vi "Receiver_Example - 2 Channel - Experiment_12.vi"() -> ()   [LabVIEW 2022 SP3]
uses:
  <vilib>/httpClient/LabVIEWHTTPClient.lvlib
panel:
  out "BER LP3":dbl
  out "BER HP3":dbl
  out "Inst. BER LP - CH1":dbl format="%#_4g"
  out "OutputHPCH0":i8[](array[numeric])
  out "BER 16QAM":dbl
  out "LP - CH0":dbl format="%#_4g"
  in  "url 2":string="http://Cobot280-02.local:5000"
  out "Numeric":i32
  out "HP - CH0":dbl format="%#_4g"
  in  "url":string="http://Cobot280-01.local:5000"
  out "x = 0?":bool
  out "iterationsIM":dbl
  in  "State":i32
  in  "Counter":dbl
  in  "Tab Control 3":enum32{"OFDM - 4QAM", "16QAM"}(tab)
  in  "Switch mode":bool
  in  "Tab Control":T1(tab)
  in  "USRP ControledParameters":T2={"Active Antenna"="RX2", "Gain (dB)"=10.0, "Carrier Frequency"=2400000000.0, "IQ Rate"=2000000.0, "Active channels"="0,1"} {"IQ Rate" format="%#_6p"; "Carrier Frequency" format="%#_6p"; "Gain (dB)" format="%#_6f"}
  in  "Device selection":refnum<k15>="RIO0"
  in  "Trigger level":dbl=0.005 format="%f"
  out "CH0":T3
  out "CH1":T3
  out "SIG valid? - CH1":bool
  out "SIG valid? - CH0":bool
  out "Frequency offset - CH1":dbl
  out "Frequency offset - CH0":dbl
  out "Coerced Parameters":T4={"IQ Rate"=100000.0, "Carrier  Freq."=100000.0, "Gain"=0.0} {"Gain" format="%#_6f"; "Carrier  Freq." format="%#_6p"; "IQ Rate" format="%#_6p"}
  out "Error out":errorcluster
  out "Inst. BER HP - CH0":dbl format="%#_4g"
  out "Acc. BER HP - CH0":dbl format="%#_4g"
  out "Acum. Err HP - CH0":dbl
  out "No. Bits HP - CH0":dbl
  out "Acc. BER LP - CH0":dbl format="%#_4g"
  out "Inst. BER - CH1":dbl format="%#_4g"
  out "Inst. BER LP - CH0":dbl format="%#_4g"
  out "No. Bits - CH1":dbl
  out "No. Bits LP - CH0":dbl
  out "Acum. Err - CH1":dbl
  out "Acum. Err LP - CH0":dbl
  in  "Record BER":bool
  in  "Refresh Button":bool
  out "Acc. BER - CH1":dbl format="%#_4g"
  in  "Boolean 2":bool
  in  "Expected message HP - CH0":string="Critical Dataaaaa\nCritical Dataaaaa\nCritical Dataaaaa\nCritical Dataaaaa\nCritical Dataaaaa"
  out "Expected message HP Detected CH0":string="Non Critical Data\nNon Critical Data\nNon Critical Data\nNon Critical Data\nNon Critical Data"
  in  "Boolean 3":bool
  in  "Boolean":bool
  out "Expected message HP Detected CH1":string="Non Critical Data\nNon Critical Data\nNon Critical Data\nNon Critical Data\nNon Critical Data"
  out "Expected message LP Detected CH0":string="Non Critical Data\nNon Critical Data\nNon Critical Data\nNon Critical Data\nNon Critical Data"
  in  "Expected message - CH1":string="Critical Dataaaaa\nCritical Dataaaaa\nCritical Dataaaaa\nCritical Dataaaaa\nCritical Dataaaaa"
  in  "Expected message LP - CH0":string="Non Critical Data\nNon Critical Data\nNon Critical Data\nNon Critical Data\nNon Critical Data"
  in  "Boolean 5":bool
  in  "Expected message LP - CH1":string="Non Critical Data\nNon Critical Data\nNon Critical Data\nNon Critical Data\nNon Critical Data"
  out "Expected message LP Detected CH1":string="Non Critical Data\nNon Critical Data\nNon Critical Data\nNon Critical Data\nNon Critical Data"
  in  "High-Power Window Size":dbl=15.0 format="%#_6p"
  in  "Low-Power Window Size - CH0":dbl=15.0 format="%#_6p"
  in  "Threshold":dbl=10.0
  in  "Channel":bool
  in  "Expected message HP - CH0 2":string="Critical Dataaaaa\nCritical Dataaaaa\nCritical Dataaaaa\nCritical Dataaaaa\nCritical Dataaaaa\nNon Critical Data\nNon Critical Data\nNon Critical Data\nNon Critical Data\nNon Critical Data"
  in  "Tab Control 2":enum32{"1 Channel", "2 Channel"}(tab)
  in  "Save data 1 channel":bool
  out "Constellation Map 1 Channel":cdb[](graph)
  out "Low-Power BER - 1 Channel":dbl(graph)
  out "High-Power BER - 1 Channel":dbl(graph)
  out "High-Power Decoded message - 1 Channel":string
  out "Low-Power Decoded message - 1 Channel":string
  in  "Color Box":u32(colorbox)=11025761
  in  "Color Box 2":u32(colorbox)=7377308
  out "Low-Power Decoded message - CH0":string
  out "Decoded message - CH1":string
  out "Constellation Map 2 Channel":cluster{"Constellation":cdb[]}[](graph)
  out "Low-Power BER - 2 Channels":T5(graph)
  out "High-Power BER":T6(graph)
  out "High-Power Decoded message - CH0":string
  out "Low-Power Decoded message - CH1":string
  out "CH1 2":bool
  out "CH0 2":bool
  in  "Save data 2 channels":bool
  in  "Color Box 3":u32(colorbox)=11025761
  in  "Color Box 4":u32(colorbox)=7377308
  in  "Save data":bool
  out "Expected message  HP  Detected 2":string="Critical Dataaaaa\nCritical Dataaaaa\nCritical Dataaaaa\nCritical Dataaaaa\nCritical Dataaaaa"
  in  "Boolean 4":bool
  in  "High-Power Window Size 2":dbl=15.0 format="%#_6p"
  out "High-Power Instantaneous BER Graph 2":u8(slide) scale=0.0..100.0
  out "High-Power BER Graph 2":dbl(graph)
  out "No. Bits HP 2":dbl
  out "Acc. BER  HP 2":dbl format="%#_4g"
  out "Acum. Err HP 2":dbl
  out "Inst. BER HP 2":dbl format="%#_4g"
  in  "Expected message 2 HP 2":string="Critical Dataaaaa\nCritical Dataaaaa\nCritical Dataaaaa\nCritical Dataaaaa\nCritical Dataaaaa"
  out "High-Power Decoded Message 2":string
  in  "Record BER 2":bool
  out "Constellation Map 2":cdb[](graph)
  out "Frequency offset 2":dbl
  out "SIG valid? 2":bool
  in  "Refresh Button 2":bool
  out "Error out 2":errorcluster
  in  "error in (no error)":errorcluster
  # "OFDM Superposition Coded Receiver"
  # "Superposition coded\n(criticality-aware)"
  # "Single stream\n(criticality-agnostic)"
  # "1 Channel"
  # "2 Channel"
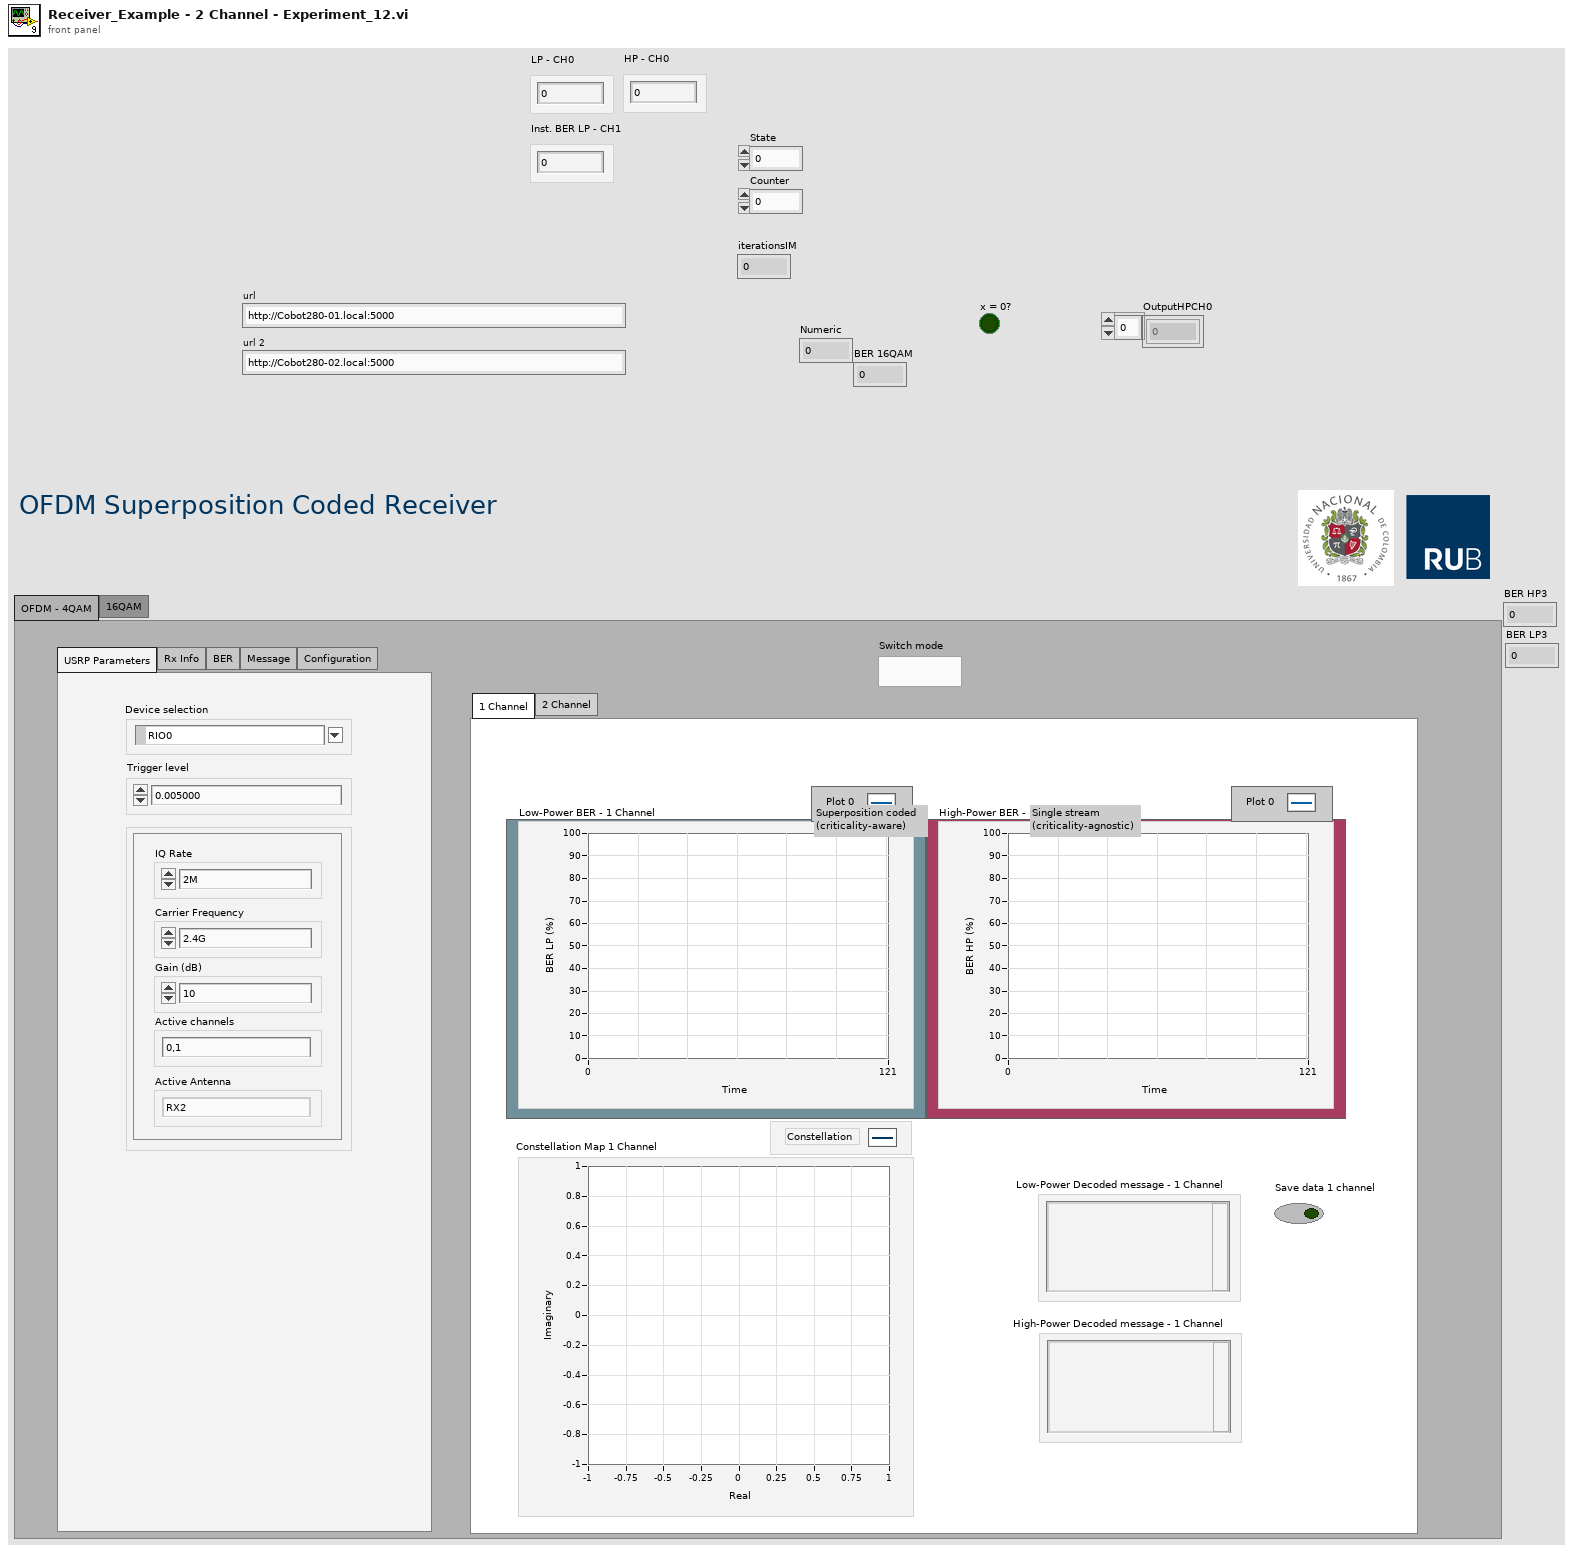
[diagram p1: front panel]
types:
  T1 = enum32{"USRP Parameters", "Rx Info", "BER", "Message", "Configuration"}
  T2 = cluster{"Active Antenna":string, "Gain (dB)":dbl, "Carrier Frequency":dbl, "IQ Rate":dbl, "Active channels":string}
  T3 = cluster{"Modulation type":enum16{"QPSK(4QAM)", "64QAM", "16QAM", "BPSK"}, "BCC rate (k/n)":enum16{"1/2", "2/3", "3/4"}}
  T4 = cluster{"IQ Rate":dbl, "Carrier  Freq.":dbl, "Gain":dbl}
  T5 = cluster{"Graph Instantaneous BER":dbl, "Graph Instantaneous BER":dbl, "Graph Instantaneous BER":dbl}
  T6 = cluster{"Graph Instantaneous BER":dbl, "Graph Instantaneous BER":dbl, "Inst. BER - CH1":dbl}
  T7 = enum16{"open", "replace", "create", "open or create", "replace or create", "replace or create with confirmation"}
  T8 = cluster{"coerced IQ rate":dbl, "coerced carrier frequency":dbl, "coerced gain":dbl}
  T9 = typedef "LabVIEWHTTPClient.lvlib/ClientHandle.ctl" = refnum<k1>
  T10 = typedef "angle_speed_def.ctl" = cluster{"degrees":dbl[], "speed":i32}
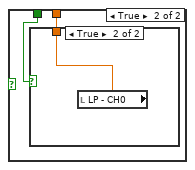
[diagram p2: hidden frame]
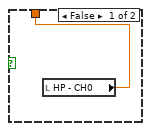
[diagram p3: hidden frame]
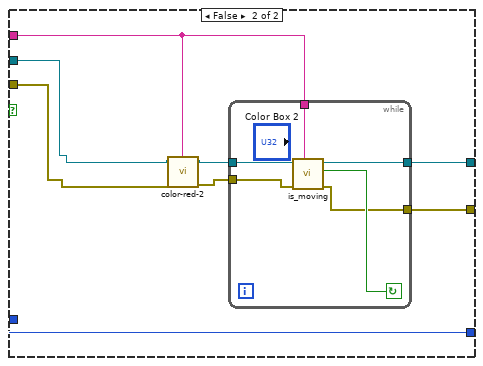
[diagram p4: hidden frame]
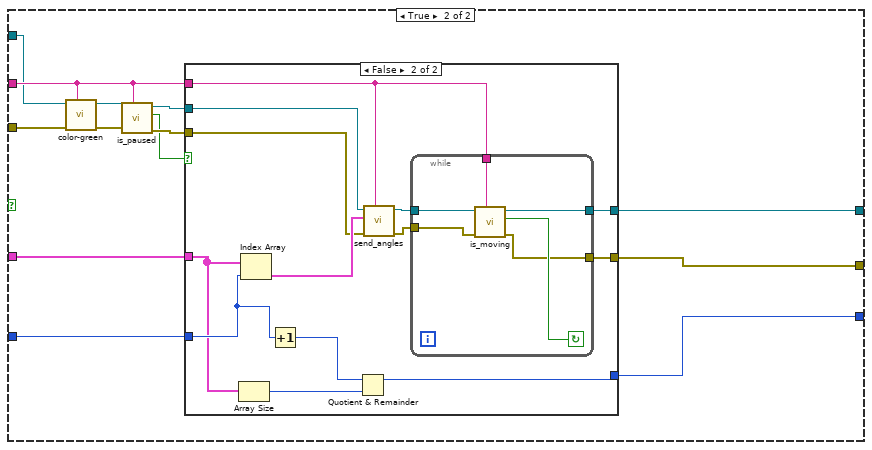
[diagram p5: hidden frame]
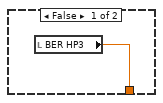
[diagram p7: hidden frame]
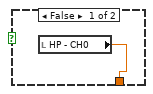
[diagram p8: hidden frame]
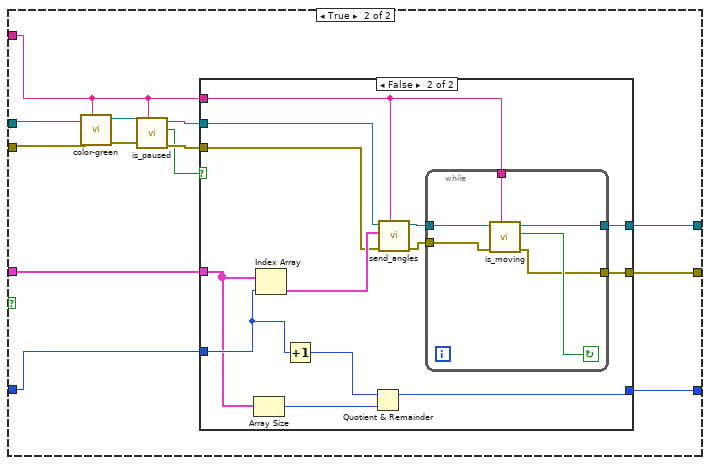
[diagram p10: hidden frame]
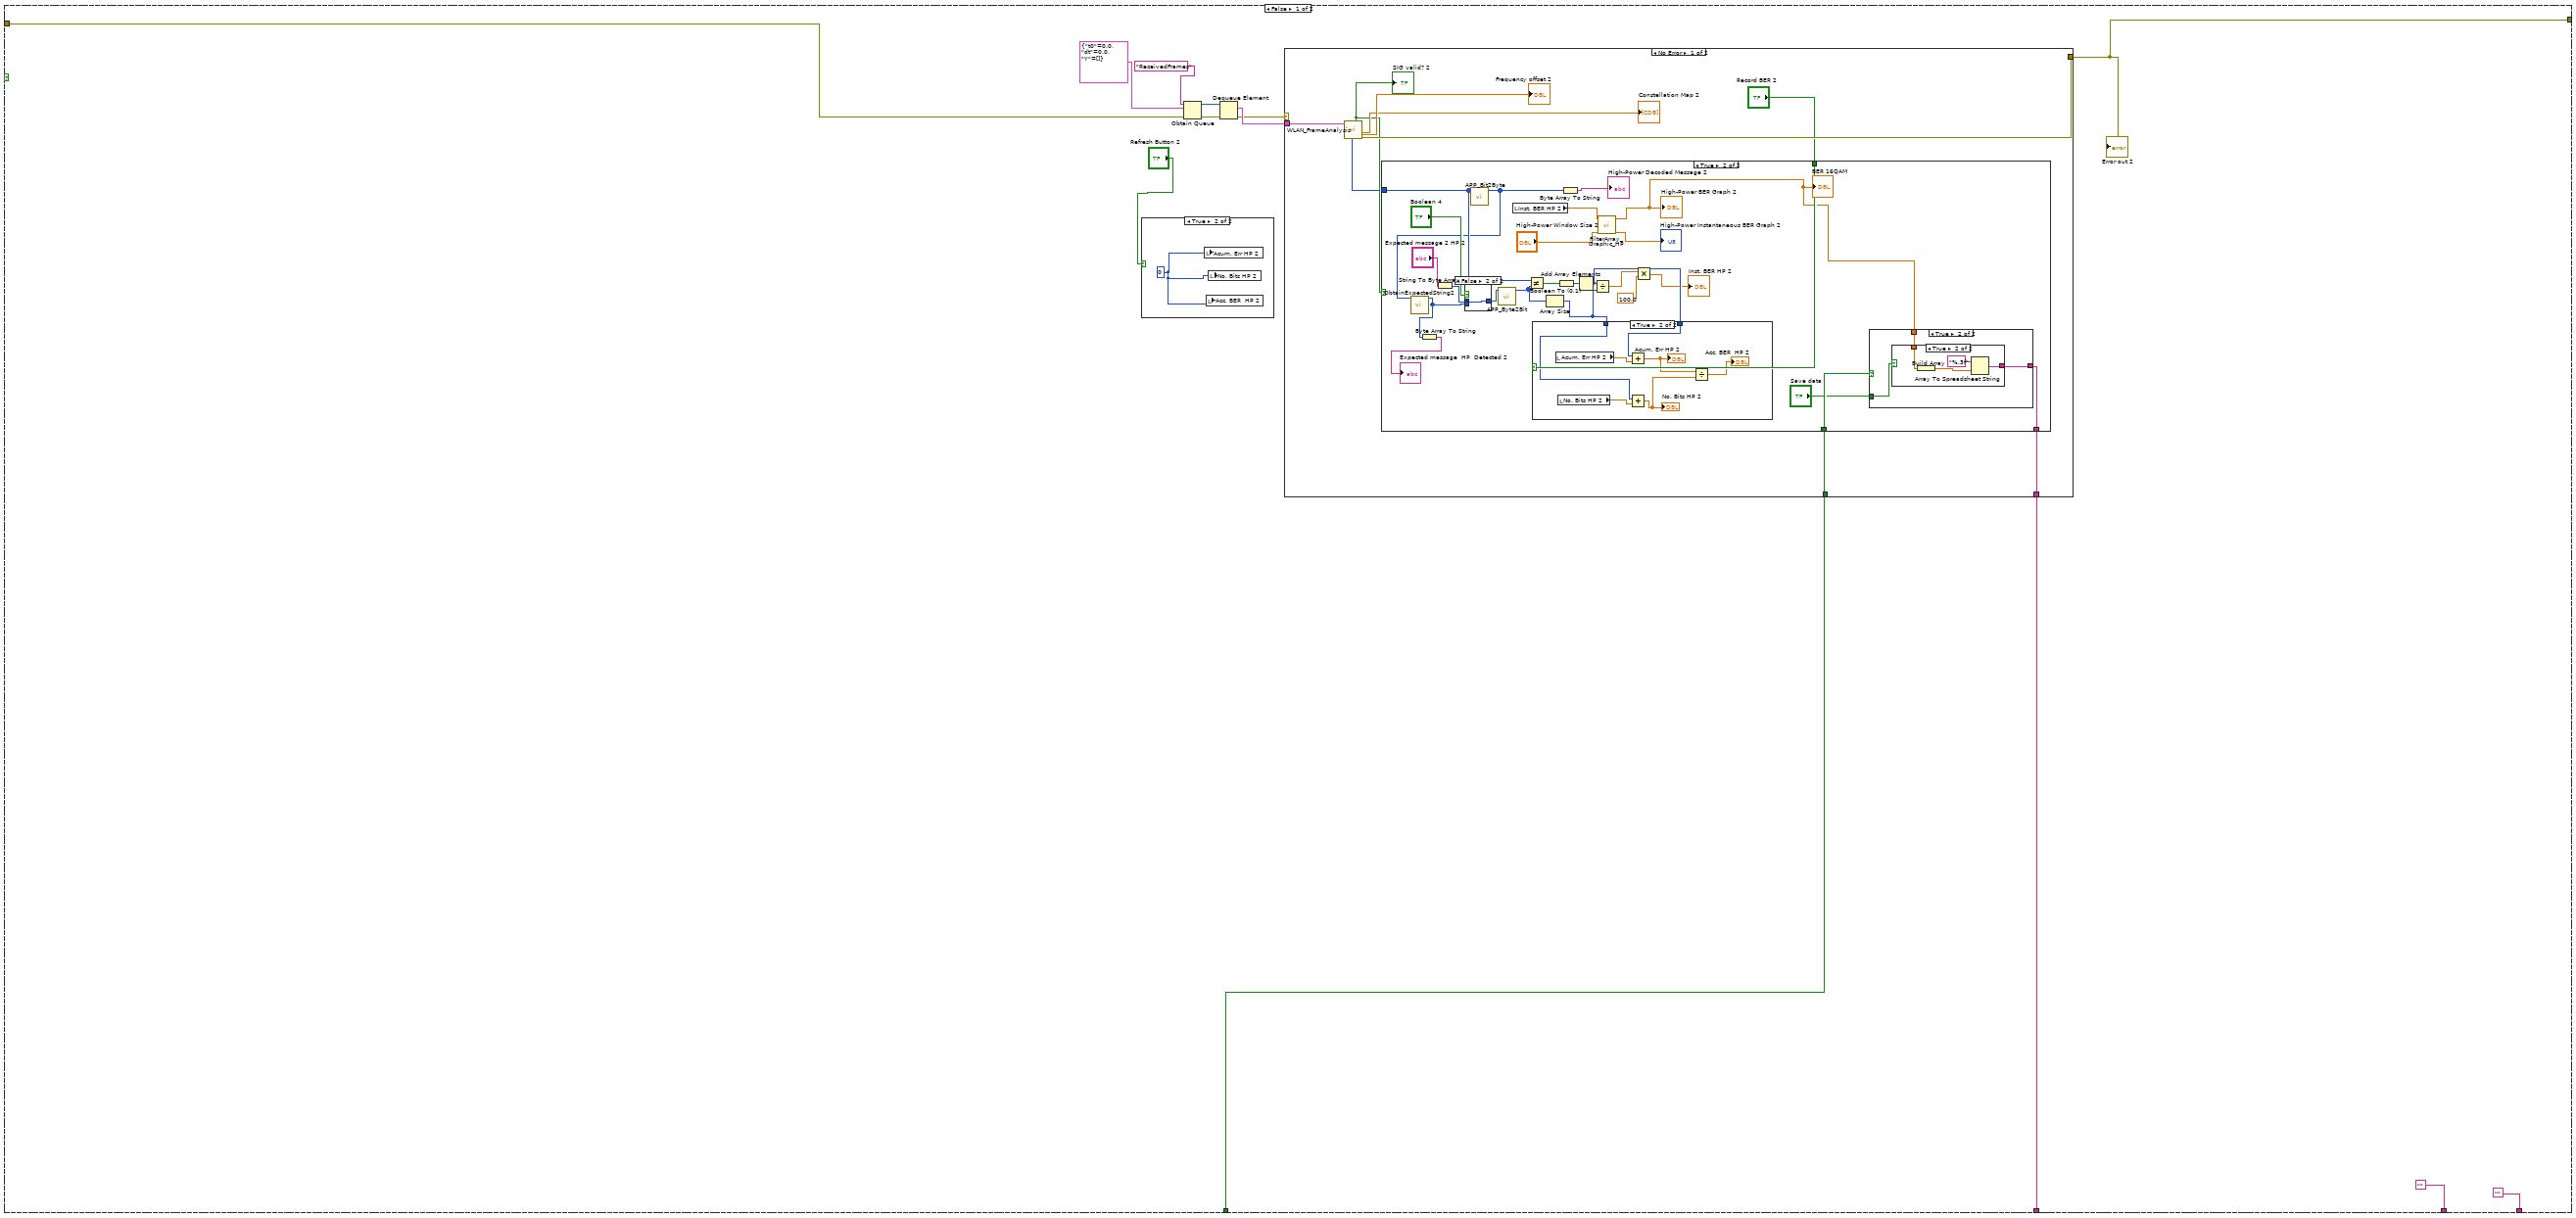
[diagram p12: hidden frame]
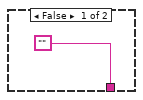
[diagram p14: hidden frame]
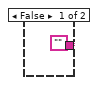
[diagram p15: hidden frame]
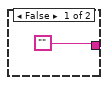
[diagram p16: hidden frame]
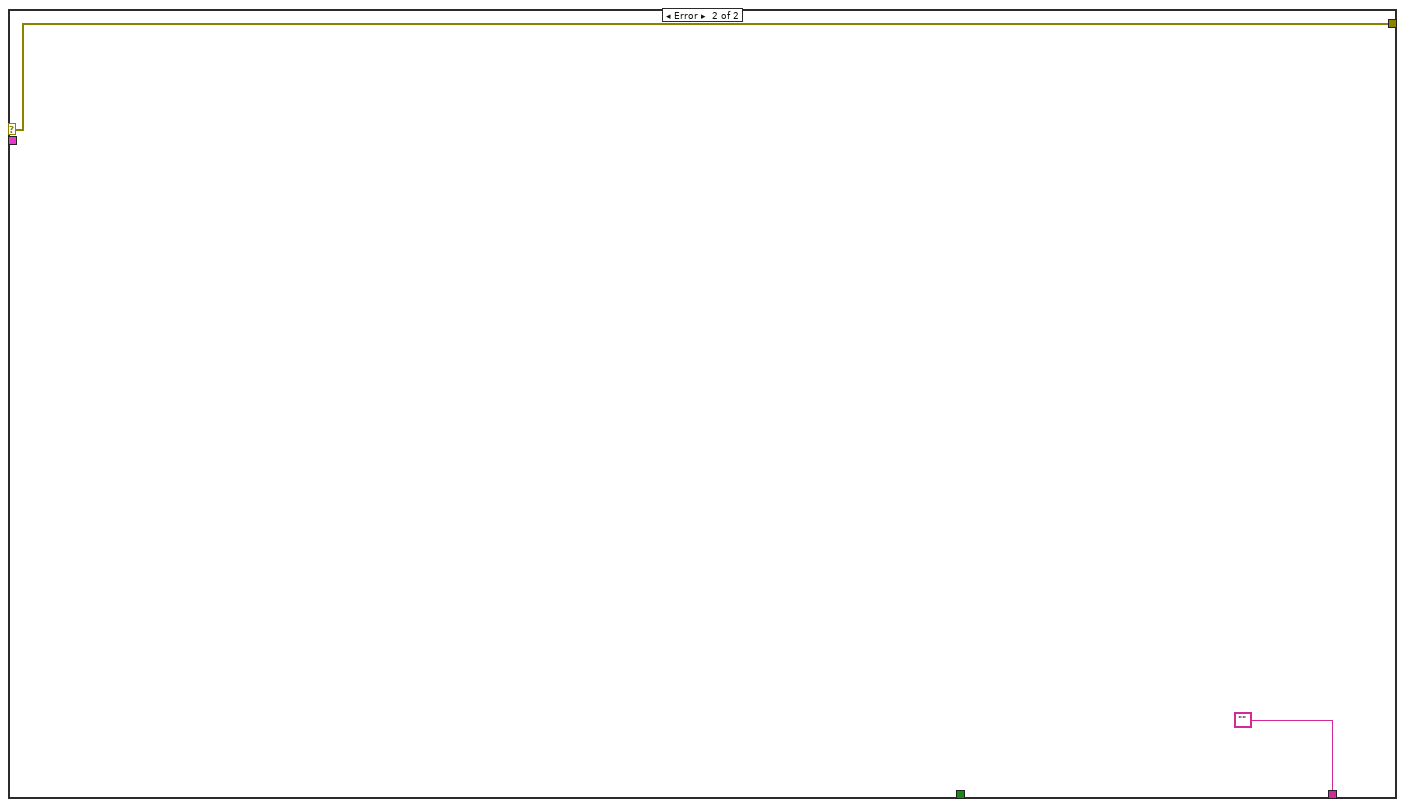
[diagram p19: hidden frame]
diagram:
  w23 = path "C:/Users/DKS/Desktop/Experiment/23_11_2023_with_graphs/12.10.2023/Supercoded Receiver with BER 12.10.2023/OFDM-Framework-LabVIEW-master/data"
  w45 = 0
  n1 = Build Path(base path=w23, name or relative path=path "data_OneChannel.txt" ("default name")) -> (appended path=w33:path)
  n2 = Build Path(base path=w23, name or relative path=path "data_16QAM.txt" ("default name")) -> (appended path=w43:path)
  n3 = Build Path(base path=w23, name or relative path=path "data_TwoChannels.txt" ("default name")) -> (appended path=w28:path)
  n4 = Delete(path (use dialog)=w33) -> (deleted path=w32:path)  [unwired: 4 in, 2 out]
  n5 = Delete(path (use dialog)=w43) -> (deleted path=w42:path)  [unwired: 4 in, 2 out]
  n6 = call "USRP_RXInit.vi"("device names"="Device selection", "USRP ControledParameters"="USRP ControledParameters", "error in (no error)"="error in (no error)") -> ("session handle out"=w48:refnum<k15>, "USRP CoercedParamters"=→"Coerced Parameters":T8, "error out"=w51:errorcluster)  [unwired: 5 in]
  n7 = Delete(path (use dialog)=w28) -> (deleted path=w27:path)  [unwired: 4 in, 2 out]
  n8 = Open/Create/Replace File(file path (use dialog)=w32, operation (0:open)=T7."create", access (0:read/write)=enum16{"read/write", "read-only", "write-only"}."write-only") -> (refnum out=w20:refnum<file>, error out=w19:errorcluster)  [unwired: 1 in, 3 out]
  n9 = Open/Create/Replace File(file path (use dialog)=w42, operation (0:open)=T7."create", access (0:read/write)=enum16{"read/write", "read-only", "write-only"}."write-only") -> (refnum out=w36:refnum<file>, error out=w37:errorcluster)  [unwired: 1 in, 3 out]
  n10 = Open/Create/Replace File(file path (use dialog)=w27, operation (0:open)=T7."create", access (0:read/write)=enum16{"read/write", "read-only", "write-only"}."write-only") -> (refnum out=w18:refnum<file>, error out=w17:errorcluster)  [unwired: 1 in, 3 out]
  n11 = call "WLAN_FrameCapture - 2 Channels.vi"("error in (no error)"=w51, "Trigger level"="Trigger level", "session handle"=w48) -> ()  [unwired: 8 in]
  n12 = while {
    tunnel: w51 -> [w77]
    tunnel: [w76] -> w49
    shift-right: [w71] -> w35
    shift-left: w37 -> [w69]
    shift-right: [w70] -> w34
    shift-left: w36 -> [w68]
    shift-right: [w65] -> w16
    shift-left: w20 -> [w66]
    shift-right: [w63] -> w15
    shift-left: w19 -> [w64]
    shift-right: [w59] -> w14
    shift-left: w18 -> [w62]
    shift-right: [w60] -> w13
    shift-left: w17 -> [w61]
    i -> [w56]
    stop <- FALSE stop-if-true
    n13 = Not(x="Switch mode") -> ()  [unwired: 1 out]
    n14 = Quotient & Remainder(x=w56, y=1) -> (x-y*floor(x/y)=w73:i32)  [unwired: 1 out]
    n15 = Equal To 0?(x=w73) -> (x = 0?=w72:bool)
    "x = 0?" <- w72
    n16 = case shown="True" TRUE {
      tunnel: w77 -> [w83 w169]
      tunnel: [w82 w168] -> w76
      tunnel: w72 -> [w81 w164]
      tunnel: [w80 ""] -> w67
      tunnel: ["" w163] -> w58
      tunnel: ["" w161] -> w57
      frame False {
        n17 = case shown="True" "Refresh Button 2" {
          frame False {
          }
          frame True {
            w91 = 0
            n18 = local write "Acum. Err HP 2"(w91) -> ()
            n19 = local write "Acc. BER  HP 2"(w91) -> ()
            n20 = local write "No. Bits HP 2"(w91) -> ()
          }
        }
        n21 = Obtain Queue(name (unnamed)="ReceivedFrames", element data type=cluster{"t0":dbl, "dt":dbl, "Y":cdb[]} {"t0"=0.0, "dt"=0.0, "Y"=[]} ("data"), error in (no error)=w83) -> (queue out=w84:refnum<queue>, error out=w87:errorcluster)  [unwired: 2 in, 1 out]
        n22 = Dequeue Element(queue=w84, error in (no error)=w87) -> (element=w86:cluster{"t0":dbl, "dt":dbl, "Y":cdb[]}, error out=w85:errorcluster)  [unwired: 1 in, 2 out]
        n23 = case shown="No Error" w85 {
          selector: w85 -> [_ w146]
          tunnel: w86 -> [w99 _]
          tunnel: [w100 w146] -> w82
          tunnel: w81 -> [w93 _]
          tunnel: [w92 ""] -> w80
          frame No Error {
            n24 = call "WLAN_FrameAnalysis.vi"("input cluster"=w99) -> ("error out"=w100:errorcluster, "Constellation"=→"Constellation Map 2":cdb[], "Frequency offset"=→"Frequency offset 2":dbl, "SIG valid?"=w95:bool, "outputbitsHP"=w94:i8[])  [unwired: 4 in, 2 out]
            "SIG valid? 2" <- w95
            n25 = case shown="True" w95 {
              tunnel: "Record BER 2" -> [_ w120]
              tunnel: w94 -> [_ w115]
              tunnel: w93 -> [_ w105]
              tunnel: ["" w103] -> w92
              frame False {
              }
              frame True {
                n26 = String To Byte Array(string="Expected message 2 HP 2") -> (unsigned byte array=w113:u8[])
                n27 = call "APP_Bit2Byte.vi"("input bit stream"=w115) -> ("output byte stream"=w109:u8[])  [unwired: 10 in]
                n28 = call "ObtainExpectedString2.vi"("Array"=w109) -> ("detectedMessage"=w111:i8[])  [unwired: 9 in]
                n29 = Byte Array To String(unsigned byte array=w111) -> (string=→"Expected message  HP  Detected 2":string)
                n30 = case shown="False" "Boolean 4" {
                  tunnel: [w136 w137] -> w114
                  tunnel: w113 -> [_ w137]
                  tunnel: w111 -> [w136 _]
                  frame True {
                  }
                  frame False {
                  }
                }
                n31 = call "APP_Byte2Bit.vi"("input byte stream"=w114) -> ("output bit stream"=w116:i8[])  [unwired: 10 in]
                n32 = local read "Inst. BER HP 2"() -> (w119:dbl)
                n33 = Not Equal?(x=w115, y=w116) -> (x != y?=w124:bool[])
                n34 = Array Size(array=w116) -> (size(s)=w121:i32)
                n35 = Boolean To (0,1)(Boolean=w124) -> (0, 1=w123:i16[])
                n36 = Byte Array To String(unsigned byte array=w109) -> (string=→"High-Power Decoded Message 2":string)
                n37 = Add Array Elements(numeric array=w123) -> (sum=w122:i16)
                n38 = case shown="True" w120 {
                  tunnel: w122 -> [_ w143]
                  tunnel: w121 -> [_ w138]
                  frame False {
                  }
                  frame True {
                    n39 = local read "Acum. Err HP 2"() -> (w144:dbl)
                    n40 = local read "No. Bits HP 2"() -> (w140:dbl)
                    n41 = Add(x=w143, y=w144) -> (x+y=w142:dbl)
                    "Acum. Err HP 2" <- w142
                    n42 = Add(x=w138, y=w140) -> (x+y=w139:dbl)
                    "No. Bits HP 2" <- w139
                    n43 = Divide(x=w142, y=w139) -> (x/y=→"Acc. BER  HP 2":dbl)
                  }
                }
                n44 = Divide(x=w122, y=w121) -> (x/y=w108:dbl)
                n45 = call "FilterArray_Graphic_HP.vi"("Window Size"="High-Power Window Size 2", "Instantaneous BER"=w119) -> ("Slide Bar"=→"High-Power Instantaneous BER Graph 2":dbl, "Graph Instantaneous BER"=w102:dbl)  [unwired: 4 in]
                "High-Power BER Graph 2" <- w102
                "BER 16QAM" <- w102
                n46 = Multiply(x=w108, y=100.0) -> (x*y=→"Inst. BER HP 2":dbl)
                n47 = case shown="True" w105 {
                  tunnel: ["" w130] -> w103
                  tunnel: w102 -> [_ w129]
                  tunnel: "Save data" -> [_ w128]
                  frame False {
                  }
                  frame True {
                    n48 = case shown="True" w128 {
                      tunnel: ["" w133] -> w130
                      tunnel: w129 -> [_ w132]
                      frame False {
                      }
                      frame True {
                        n49 = Build Array(w132) -> (w135:dbl[])
                        n50 = Array To Spreadsheet String(array=w135, 3:"%.3f") -> (spreadsheet string=w133:string)  [unwired: 1 out]
                      }
                    }
                  }
                }
              }
            }
          }
          frame Error {
          }
        }
        "Error out 2" <- w82
      }
      frame True {
        w204 = cluster{"t0":dbl, "dt":dbl, "Y":cdb[]} {"t0"=0.0, "dt"=0.0, "Y"=[]} ("data")
        n51 = Obtain Queue(name (unnamed)="ReceivedFrames", element data type=w204, error in (no error)=w169) -> (queue out=w170:refnum<queue>, error out=w172:errorcluster)  [unwired: 2 in, 1 out]
        n52 = Obtain Queue(name (unnamed)="ReceivedFrames_1", element data type=w204, error in (no error)=w169) -> (queue out=w174:refnum<queue>, error out=w175:errorcluster)  [unwired: 2 in, 1 out]
        n53 = Dequeue Element(queue=w170, error in (no error)=w172) -> (element=w171:cluster{"t0":dbl, "dt":dbl, "Y":cdb[]}, error out=w178:errorcluster)  [unwired: 1 in, 2 out]
        n54 = Dequeue Element(queue=w174, error in (no error)=w175) -> (element=w180:cluster{"t0":dbl, "dt":dbl, "Y":cdb[]}, error out=w184:errorcluster)  [unwired: 1 in, 2 out]
        n55 = Not(x="Channel") -> (.not. x?=w165:bool)
        n56 = Merge Errors(w178, w184) -> (w177:errorcluster)
        n57 = case shown="No Error" w177 {
          tunnel: w171 -> [w380 _]
          tunnel: w177 -> [_ w480]
          tunnel: w178 -> [w377 _]
          tunnel: [w376 dbl[] []] -> w195
          tunnel: [w375 w480] -> w181
          tunnel: "Record BER" -> [w374 _]
          tunnel: "Record BER" -> [w373 _]
          tunnel: w165 -> [w372 _]
          frame No Error {
            n58 = local read "Switch mode"() -> (w371:bool)
            n59 = call "WLAN_FrameAnalysis.vi"("error in (no error)"=w377, "input cluster"=w380) -> ("error out"=w375:errorcluster, "Constellation"=w376:cdb[], "Modulation parameter"=w381:T3, "output bits"=w382:i8[], "Frequency offset"=→"Frequency offset - CH0":dbl, "SIG valid?"=w378:bool, "outputbitsHP"=w379:i8[])  [unwired: 3 in]
            "SIG valid? - CH0" <- w378
            n60 = Not(x=w371) -> (.not. x?=w370:bool)
            n61 = case shown="True" w378 {
              tunnel: w382 -> [_ w435]
              tunnel: w381 -> [_ w455]
              tunnel: w373 -> [_ w452]
              tunnel: w372 -> [_ w438]
              tunnel: w370 -> [_ w436]
              frame False {
              }
              frame True {
                n62 = case shown="False" w436 {
                  tunnel: w435 -> [_ w465]
                  tunnel: [w463 w465] -> w437
                  frame False {
                    n63 = local read "OutputHPCH0"() -> (w462:i8[])
                    n64 = Array Size(array=w462) -> (size(s)=w461:i32)
                    n65 = Divide(x=w461, y=2) -> (x/y=w458:dbl)
                    n66 = Add(x=4.0, y=w458) -> (x+y=w460:dbl)
                    n67 = Subtract(x=w458, y=5.0) -> (x-y=w456:dbl)
                    n68 = Array Subset(array=w462, index=w460, length=w456) -> (w463:i8[])
                  }
                  frame True {
                  }
                }
                n69 = String To Byte Array(string="Expected message LP - CH0") -> (unsigned byte array=w445:u8[])
                n70 = call "APP_Bit2Byte.vi"("input bit stream"=w437) -> ("output byte stream"=w444:u8[])  [unwired: 10 in]
                n71 = call "ObtainExpectedString.vi"("Array"=w444) -> ("detectedMessage"=w443:i8[])  [unwired: 9 in]
                n72 = Byte Array To String(unsigned byte array=w443) -> (string=→"Expected message LP Detected CH0":string)
                n73 = case shown="False" "Boolean" {
                  tunnel: [w470 w471] -> w447
                  tunnel: w445 -> [_ w471]
                  tunnel: w443 -> [w470 _]
                  frame True {
                  }
                  frame False {
                  }
                }
                n74 = call "APP_Byte2Bit.vi"("input byte stream"=w447) -> ("output bit stream"=w446:i8[])  [unwired: 10 in]
                n75 = Not Equal?(x=w435, y=w446) -> (x != y?=w453:bool[])
                n76 = Array Size(array=w446) -> (size(s)=w451:i32)
                n77 = Boolean To (0,1)(Boolean=w453) -> (0, 1=w454:i16[])
                n78 = Add Array Elements(numeric array=w454) -> (sum=w450:i16)
                n79 = case shown="True" w452 {
                  tunnel: w451 -> [_ w477]
                  tunnel: w450 -> [_ w475]
                  frame False {
                  }
                  frame True {
                    n80 = local read "Acum. Err LP - CH0"() -> (w476:dbl)
                    n81 = local read "No. Bits LP - CH0"() -> (w478:dbl)
                    n82 = Add(x=w477, y=w478) -> (x+y=w474:dbl)
                    n83 = Add(x=w475, y=w476) -> (x+y=w473:dbl)
                    "Acum. Err LP - CH0" <- w473
                    n84 = local write "No. Bits LP - CH0"(w474) -> ()
                    n85 = Divide(x=w473, y=w474) -> (x/y=→"Acc. BER LP - CH0":dbl)
                  }
                }
                n86 = Divide(x=w450, y=w451) -> (x/y=w449:dbl)
                n87 = Multiply(x=w449, y=100.0) -> (x*y=→"Inst. BER LP - CH0":dbl)
                n88 = Byte Array To String(unsigned byte array=w444) -> (string=w441:string)
                n89 = case shown="True" w438 {
                  tunnel: w441 -> [w467 w469]
                  tunnel: ["" ("string") w469] -> w440
                  tunnel: [w467 "" ("string")] -> w439
                  frame False {
                  }
                  frame True {
                  }
                }
                "Low-Power Decoded message - CH0" <- w439
                "Low-Power Decoded message - 1 Channel" <- w440
                "CH0" <- w455
              }
            }
            n90 = case shown="True" w378 {
              tunnel: w379 -> [_ w388]
              tunnel: w374 -> [_ w404]
              tunnel: w372 -> [_ w393]
              tunnel: w370 -> [_ w391]
              frame False {
              }
              frame True {
                n91 = String To Byte Array(string="Expected message HP - CH0") -> (unsigned byte array=w390:u8[])
                n92 = case shown="False" w391 {
                  tunnel: w388 -> [w414 w418]
                  tunnel: [w415 w418] -> w392
                  tunnel: [w407 w417] -> w387
                  tunnel: w390 -> [_ w417]
                  frame False {
                    n93 = Array Size(array=w414) -> (size(s)=w411:i32)
                    n94 = Divide(x=w411, y=2) -> (x/y=w410:dbl)
                    n95 = Subtract(x=w410, y=5) -> (x-y=w412:dbl)
                    n96 = Array Subset(array=w414, index=0, length=w412) -> (w415:i8[])
                    n97 = String To Byte Array(string="Expected message HP - CH0 2") -> (unsigned byte array=w407:u8[])
                  }
                  frame True {
                  }
                }
                n98 = call "APP_Byte2Bit.vi"("input byte stream"=w387) -> ("output bit stream"=w389:i8[])  [unwired: 10 in]
                n99 = Not Equal?(x=w388, y=w389) -> (x != y?=w405:bool[])
                n100 = Array Size(array=w389) -> (size(s)=w403:i32)
                n101 = Boolean To (0,1)(Boolean=w405) -> (0, 1=w406:i16[])
                n102 = Add Array Elements(numeric array=w406) -> (sum=w402:i16)
                n103 = case shown="True" w404 {
                  tunnel: w403 -> [_ w430]
                  tunnel: w402 -> [_ w428]
                  frame False {
                  }
                  frame True {
                    n104 = local read "Acum. Err HP - CH0"() -> (w429:dbl)
                    n105 = local read "No. Bits HP - CH0"() -> (w431:dbl)
                    n106 = Add(x=w430, y=w431) -> (x+y=w427:dbl)
                    n107 = local write "No. Bits HP - CH0"(w427) -> ()
                    n108 = Add(x=w428, y=w429) -> (x+y=w426:dbl)
                    "Acum. Err HP - CH0" <- w426
                    n109 = Divide(x=w426, y=w427) -> (x/y=→"Acc. BER HP - CH0":dbl)
                  }
                }
                n110 = Divide(x=w402, y=w403) -> (x/y=w401:dbl)
                n111 = call "APP_Bit2Byte.vi"("input bit stream"=w392) -> ("output byte stream"=w399:u8[])  [unwired: 10 in]
                n112 = call "ObtainExpectedString2.vi"("Array"=w399) -> ("detectedMessage"=w398:i8[])  [unwired: 9 in]
                n113 = Byte Array To String(unsigned byte array=w398) -> (string=→"Expected message HP Detected CH0":string)
                n114 = case shown="False" "Boolean 2" {
                  tunnel: [w423 w424] -> _
                  tunnel: w390 -> [_ w424]
                  tunnel: w398 -> [w423 _]
                  frame True {
                  }
                  frame False {
                  }
                }
                n115 = Multiply(x=w401, y=100.0) -> (x*y=→"Inst. BER HP - CH0":dbl)
                n116 = Byte Array To String(unsigned byte array=w399) -> (string=w394:string)
                n117 = case shown="False" w393 {
                  tunnel: w394 -> [w420 w422]
                  tunnel: ["" ("string") w422] -> w395
                  tunnel: [w420 "" ("string")] -> w396
                  frame False {
                  }
                  frame True {
                  }
                }
                "High-Power Decoded message - CH0" <- w396
                "High-Power Decoded message - 1 Channel" <- w395
                "OutputHPCH0" <- w388
              }
            }
          }
          frame Error {
          }
        }
        n118 = case shown="No Error" w184 {
          tunnel: w180 -> [w307 _]
          tunnel: "Record BER" -> [w306 _]
          tunnel: [w305 w369] -> w182
          tunnel: [w304 dbl[] []] -> w183
          tunnel: w184 -> [w303 w369]
          tunnel: w165 -> [w300 _]
          frame No Error {
            n119 = call "WLAN_FrameAnalysis.vi"("error in (no error)"=w303, "input cluster"=w307) -> ("error out"=w305:errorcluster, "Constellation"=w304:cdb[], "Modulation parameter"=w310:T3, "output bits"=w302:i8[], "Frequency offset"=→"Frequency offset - CH1":dbl, "SIG valid?"=w301:bool, "outputbitsHP"=w308:i8[])  [unwired: 3 in]
            "SIG valid? - CH1" <- w301
            n120 = case shown="True" "Refresh Button" {
              frame False {
              }
              frame True {
                w335 = 0
                n121 = local write "Acum. Err HP - CH0"(w335) -> ()
                n122 = local write "Acc. BER HP - CH0"(w335) -> ()
                n123 = local write "Acum. Err LP - CH0"(w335) -> ()
                n124 = local write "No. Bits LP - CH0"(w335) -> ()
                n125 = local write "No. Bits HP - CH0"(w335) -> ()
                n126 = local write "Acc. BER LP - CH0"(w335) -> ()
                n127 = local write "Acum. Err - CH1"(w335) -> ()
                n128 = local write "No. Bits - CH1"(w335) -> ()
                n129 = local write "Acc. BER - CH1"(w335) -> ()
              }
            }
            n130 = case shown="True" w301 {
              tunnel: w302 -> [_ w313]
              tunnel: w300 -> [_ w328]
              frame False {
              }
              frame True {
                n131 = call "APP_Bit2Byte.vi"("input bit stream"=w313) -> ("output byte stream"=w323:u8[])  [unwired: 10 in]
                n132 = call "ObtainExpectedString4.vi"("Array"=w323) -> ("detectedMessage"=w324:i8[])  [unwired: 9 in]
                n133 = Byte Array To String(unsigned byte array=w324) -> (string=→"Expected message LP Detected CH1":string)
                n134 = String To Byte Array(string="Expected message LP - CH1") -> (unsigned byte array=w327:u8[])
                n135 = case shown="False" "Boolean 5" {
                  tunnel: [w331 w332] -> w322
                  tunnel: w327 -> [_ w332]
                  tunnel: w324 -> [w331 _]
                  frame True {
                  }
                  frame False {
                  }
                }
                n136 = call "APP_Byte2Bit.vi"("input byte stream"=w322) -> ("output bit stream"=w314:i8[])  [unwired: 10 in]
                n137 = Byte Array To String(unsigned byte array=w323) -> (string=w330:string)
                n138 = Not Equal?(x=w313, y=w314) -> (x != y?=w320:bool[])
                n139 = Array Size(array=w314) -> (size(s)=w319:i32)
                n140 = case shown="True" w328 {
                  tunnel: w330 -> [w333 _]
                  tunnel: [w333 "" ("string")] -> w329
                  frame False {
                  }
                  frame True {
                  }
                }
                "Low-Power Decoded message - CH1" <- w329
                n141 = Boolean To (0,1)(Boolean=w320) -> (0, 1=w321:i16[])
                n142 = Add Array Elements(numeric array=w321) -> (sum=w318:i16)
                n143 = Divide(x=w318, y=w319) -> (x/y=w317:dbl)
                n144 = Multiply(x=w317, y=100.0) -> (x*y=→"Inst. BER LP - CH1":dbl)
              }
            }
            n145 = case shown="True" w301 {
              tunnel: w308 -> [_ w344]
              tunnel: w310 -> [_ w356]
              tunnel: w306 -> [_ w342]
              tunnel: w300 -> [_ w339]
              frame False {
              }
              frame True {
                n146 = call "APP_Bit2Byte.vi"("input bit stream"=w344) -> ("output byte stream"=w346:u8[])  [unwired: 10 in]
                n147 = call "ObtainExpectedString3.vi"("Array"=w346) -> ("detectedMessage"=w345:i8[])  [unwired: 9 in]
                n148 = Byte Array To String(unsigned byte array=w346) -> (string=w340:string)
                n149 = String To Byte Array(string="Expected message - CH1") -> (unsigned byte array=w347:u8[])
                n150 = Byte Array To String(unsigned byte array=w345) -> (string=→"Expected message HP Detected CH1":string)
                n151 = case shown="False" "Boolean 3" {
                  tunnel: [w359 w360] -> w349
                  tunnel: w347 -> [_ w360]
                  tunnel: w345 -> [w359 _]
                  frame True {
                  }
                  frame False {
                  }
                }
                n152 = call "APP_Byte2Bit.vi"("input byte stream"=w349) -> ("output bit stream"=w348:i8[])  [unwired: 10 in]
                n153 = Not Equal?(x=w344, y=w348) -> (x != y?=w354:bool[])
                n154 = Array Size(array=w348) -> (size(s)=w353:i32)
                n155 = Boolean To (0,1)(Boolean=w354) -> (0, 1=w355:i16[])
                n156 = Add Array Elements(numeric array=w355) -> (sum=w352:i16)
                n157 = case shown="True" w342 {
                  tunnel: w353 -> [_ w366]
                  tunnel: w352 -> [_ w364]
                  frame False {
                  }
                  frame True {
                    n158 = local read "No. Bits - CH1"() -> (w367:dbl)
                    n159 = local read "Acum. Err - CH1"() -> (w365:dbl)
                    n160 = Add(x=w366, y=w367) -> (x+y=w363:dbl)
                    n161 = Add(x=w364, y=w365) -> (x+y=w362:dbl)
                    "Acum. Err - CH1" <- w362
                    n162 = local write "No. Bits - CH1"(w363) -> ()
                    n163 = Divide(x=w362, y=w363) -> (x/y=→"Acc. BER - CH1":dbl)
                  }
                }
                n164 = case shown="True" w339 {
                  tunnel: w340 -> [w357 _]
                  tunnel: [w357 "" ("string")] -> w341
                  frame False {
                  }
                  frame True {
                  }
                }
                "Decoded message - CH1" <- w341
                n165 = Divide(x=w352, y=w353) -> (x/y=w350:dbl)
                n166 = Multiply(x=w350, y=100.0) -> (x*y=→"Inst. BER - CH1":dbl)
                "CH1" <- w356
              }
            }
          }
          frame Error {
          }
        }
        n167 = local read "Inst. BER LP - CH1"() -> (w153:dbl)
        n168 = local read "Inst. BER HP - CH0"() -> (w200:dbl)
        n169 = local read "Inst. BER - CH1"() -> (w191:dbl)
        n170 = Bundle("Constellation"=w195) -> (w194:cluster{"Constellation":cdb[]})  [unwired: 1 in]
        n171 = Bundle("Constellation"=w183) -> (w179:cluster{"Constellation":cdb[]})  [unwired: 1 in]
        n172 = call "FilterArray_Graphic_CH1_LP.vi"("Window Size"="Low-Power Window Size - CH0", "Instantaneous BER"=w153) -> ("Graph Instantaneous BER"=w148:dbl)  [unwired: 4 in, 1 out]
        n173 = local read "Inst. BER LP - CH0"() -> (w166:dbl)
        n174 = Equal To 0?(x="State") -> (x = 0?=w151:bool)
        n175 = Merge Errors(w181, w182) -> (w168:errorcluster)
        "Error out" <- w168
        n176 = Build Array(w194, w179) -> (w197:cluster{"Constellation":cdb[]}[])
        n177 = call "FilterArray_Graphic_CH1.vi"("Window Size"="High-Power Window Size", "Instantaneous BER"=w191) -> ("Graph Instantaneous BER"=w162:dbl)  [unwired: 4 in, 1 out]
        n178 = call "FilterArray_Graphic_HP.vi"("Window Size"="High-Power Window Size", "Instantaneous BER"=w200) -> ("Graph Instantaneous BER"=w159:dbl)  [unwired: 4 in, 1 out]
        "HP - CH0" <- w159
        n179 = case shown="0, Default" "State" {
          tunnel: "Counter" -> [w268 w288]
          tunnel: [w275 w291] -> w187
          tunnel: "Counter" -> [w263 w281]
          tunnel: [w272 w290] -> w188
          tunnel: [w270 w289] -> w160
          tunnel: w159 -> [w269 w286]
          tunnel: w162 -> [w267 w287]
          tunnel: 10.0 ("y") -> [w266 w282]
          frame 0, Default {
            n180 = Greater?(x=w269, y=10.0) -> (0:w276:bool)
            n181 = Equal?(x=w263, y=w266) -> (x = y?=w271:bool)
            n182 = Add(x=w268, y=1.0) -> (x+y=w278:dbl)
            n183 = Greater?(x=w263, y=w266) -> (0:w265:bool)
            n184 = Select(t=w278, s=w276, f=0.0) -> (s? t:f=w275:dbl)
            n185 = Select(t=w267, s=w271, f=w269) -> (s? t:f=w270:dbl)
            n186 = Select(t=1.0, s=w271, f=0.0) -> (s? t:f=w272:dbl)
            n187 = Select(t=0.0, s=w265, f=w263) -> (s? t:f=w262:dbl)
            n188 = local write "Counter"(w262) -> ()
          }
          frame 1 {
            n189 = Less?(x=w286, y=10.0) -> (x < y?=w292:bool)
            n190 = Greater?(x=w281, y=w282) -> (0:w284:bool)
            n191 = Equal?(x=w281, y=w282) -> (x = y?=w294:bool)
            n192 = Add(x=w288, y=1.0) -> (x+y=w298:dbl)
            n193 = Select(t=w298, s=w292, f=0.0) -> (s? t:f=w291:dbl)
            n194 = Select(t=0.0, s=w284, f=w281) -> (s? t:f=w285:dbl)
            n195 = local write "Counter"(w285) -> ()
            n196 = Select(t=w286, s=w294, f=w287) -> (s? t:f=w289:dbl)
            n197 = Select(t=0.0, s=w294, f=1.0) -> (s? t:f=w290:dbl)
          }
        }
        "BER HP3" <- w160
        n198 = call "FilterArray_Graphic_LP.vi"("Window Size"="Low-Power Window Size - CH0", "Instantaneous BER"=w166) -> ("Graph Instantaneous BER"=w149:dbl)  [unwired: 4 in, 1 out]
        "LP - CH0" <- w149
        n199 = Select(t=w149, s=w151, f=w148) -> (s? t:f=w147:dbl)
        "BER LP3" <- w147
        n200 = case shown="True" w165 {
          tunnel: [cdb[] [] ("Constellation") w261] -> w196
          tunnel: w195 -> [_ w261]
          tunnel: w197 -> [w259 _]
          tunnel: [w259 cluster{"Constellation":cdb[]}[] []] -> w198
          frame False {
          }
          frame True {
          }
        }
        "Constellation Map 2 Channel" <- w198
        "Constellation Map 1 Channel" <- w196
        n201 = local read "Switch mode"() -> (w158:bool)
        n202 = case shown="False" w165 {
          tunnel: w149 -> [w249 w253]
          tunnel: [nan ("Graph Instantaneous BER") w253] -> w155
          tunnel: [w250 T5 {"Graph Instantaneous BER"=nan, "Graph Instantaneous BER"=nan, "Graph Instantaneous BER"=nan}] -> w156
          tunnel: w148 -> [w248 _]
          tunnel: w147 -> [w247 _]
          frame False {
            n203 = Bundle("Graph Instantaneous BER"=w249, "Graph Instantaneous BER"=w248, "Graph Instantaneous BER"=w247) -> (w250:T5)  [unwired: 1 in]
          }
          frame True {
          }
        }
        "Low-Power BER - 2 Channels" <- w156
        n204 = Bundle("Graph Instantaneous BER"=w159, "Graph Instantaneous BER"=w162, "Graph Instantaneous BER"=w160) -> (w202:T5)  [unwired: 1 in]
        n205 = Equal To 0?(x="State") -> (x = 0?=w193:bool)
        "CH0 2" <- w193
        n206 = Not(x=w158) -> (.not. x?=w157:bool)
        n207 = Not(x=w193) -> (.not. x?=→"CH1 2":bool)
        n208 = case shown="True" w165 {
          tunnel: w159 -> [_ w257]
          tunnel: [nan w257] -> w201
          tunnel: w202 -> [w255 _]
          tunnel: [w255 T5 {"Graph Instantaneous BER"=nan, "Graph Instantaneous BER"=nan, "Graph Instantaneous BER"=nan}] -> w203
          frame False {
          }
          frame True {
          }
        }
        "High-Power BER" <- w203
        "High-Power BER - 1 Channel" <- w201
        n209 = case shown="False" w157 {
          tunnel: w155 -> [_ w206]
          tunnel: [w205 w206] -> w154
          frame False {
            n210 = local read "HP - CH0"() -> (w205:dbl)
          }
          frame True {
          }
        }
        "Low-Power BER - 1 Channel" <- w154
        n211 = local write "Counter"(w187) -> ()
        n212 = local write "State"(w188) -> ()
        n213 = case shown="True" w165 {
          tunnel: w149 -> [w211 w235]
          tunnel: w159 -> [w210 w234]
          tunnel: w164 -> [w213 w233]
          tunnel: ["" w231] -> w163
          tunnel: w162 -> [w209 _]
          tunnel: w160 -> [w208 _]
          tunnel: [w207 ""] -> w161
          frame False {
            n214 = case shown="True" w213 {
              tunnel: ["" w221] -> w207
              tunnel: w211 -> [_ w219]
              tunnel: w210 -> [_ w220]
              tunnel: "Save data 2 channels" -> [_ w218]
              tunnel: w209 -> [_ w217]
              tunnel: w208 -> [_ w216]
              frame False {
              }
              frame True {
                n215 = case shown="True" w218 {
                  tunnel: ["" w227] -> w221
                  tunnel: w219 -> [_ w226]
                  tunnel: w220 -> [_ w225]
                  tunnel: w217 -> [_ w224]
                  tunnel: w216 -> [_ w223]
                  frame False {
                  }
                  frame True {
                    n216 = Build Array(w226, w225, w224, w223) -> (w229:dbl[])
                    n217 = Array To Spreadsheet String(array=w229, 3:"%.3f") -> (spreadsheet string=w227:string)  [unwired: 1 out]
                  }
                }
              }
            }
          }
          frame True {
            n218 = case shown="True" w233 {
              tunnel: ["" w240] -> w231
              tunnel: w235 -> [_ w238]
              tunnel: w234 -> [_ w239]
              tunnel: "Save data 1 channel" -> [_ w237]
              frame False {
              }
              frame True {
                n219 = case shown="True" w237 {
                  tunnel: ["" w244] -> w240
                  tunnel: w238 -> [_ w243]
                  tunnel: w239 -> [_ w242]
                  frame False {
                  }
                  frame True {
                    n220 = Build Array(w243, w242) -> (w246:dbl[])
                    n221 = Array To Spreadsheet String(array=w246, 3:"%.3f") -> (spreadsheet string=w244:string)  [unwired: 1 out]
                  }
                }
              }
            }
          }
        }
      }
    }
    n222 = Write to Text File(file (use dialog)=w62, text=w57, error in=w61) -> (refnum out=w59:refnum<file>, error out=w60:errorcluster)  [unwired: 1 in, 1 out]
    n223 = Write to Text File(file (use dialog)=w68, text=w67, error in=w69) -> (refnum out=w70:refnum<file>, error out=w71:errorcluster)  [unwired: 1 in, 1 out]
    n224 = Write to Text File(file (use dialog)=w66, text=w58, error in=w64) -> (refnum out=w65:refnum<file>, error out=w63:errorcluster)  [unwired: 1 in, 1 out]
    "Numeric" <- w56
  }
  n225 = call <vilib>:"OpenHandle.vi"() -> ("client handle out"=w7:T9, "error out"=w8:errorcluster)  [unwired: 14 in]
  n226 = call "wave.vi"() -> ("sequenz"=w9:T10[])  [unwired: 11 in]
  n227 = call <vilib>:"OpenHandle.vi"() -> ("client handle out"=w3:T9, "error out"=w2:errorcluster)  [unwired: 14 in]
  n228 = while {
    shift-right: [w492] -> _
    shift-left: 0 -> [w493]
    tunnel: w9 -> [w491]
    tunnel: w2 -> [w490]
    tunnel: w3 -> [w489]
    tunnel: [w488] -> w6
    tunnel: [w487] -> w4
    tunnel: "Threshold" -> [w486]
    stop <- FALSE stop-if-true
    n229 = local read "Channel"() -> (w481:bool)
    n230 = Not(x=w481) -> (.not. x?=w482:bool)
    n231 = local read "Switch mode"() -> (w484:bool)
    n232 = Not(x=w484) -> (.not. x?=w483:bool)
    n233 = case shown="False" w482 {
      tunnel: [w498 w500] -> w485
      tunnel: w483 -> [_ w499]
      frame False {
        n234 = local read "BER LP3"() -> (w498:dbl)
      }
      frame True {
        n235 = case shown="True" w499 {
          tunnel: [w501 w502] -> w500
          frame False {
            n236 = local read "HP - CH0"() -> (w501:dbl)
          }
          frame True {
            n237 = local read "LP - CH0"() -> (w502:dbl)
          }
        }
      }
    }
    n238 = Wait (ms)(milliseconds to wait=u32 300) -> ()  [unwired: 1 out]
    n239 = Less?(x=w485, y=w486) -> (x < y?=w495:bool)
    n240 = case shown="False" w495 {
      tunnel: "url 2" -> [w507 w537]
      tunnel: w493 -> [w509 w536]
      tunnel: [w508 w535] -> w492
      tunnel: w491 -> [_ w534]
      tunnel: w490 -> [w504 w533]
      tunnel: w489 -> [w503 w532]
      tunnel: [w506 w531] -> w488
      tunnel: [w505 w530] -> w487
      frame False {
        n241 = call "is_paused.vi"("url"=w507, "error in (no error)"=w504, "client handle"=w503) -> ("error out"=w511:errorcluster, "paused"=w510:bool, "client handle out"=w512:T9)  [unwired: 6 in]
        n242 = case shown="True" w510 {
          tunnel: w507 -> [_ w518]
          tunnel: w511 -> [w514 w520]
          tunnel: w512 -> [w515 w519]
          tunnel: [w515 w523] -> w506
          tunnel: [w514 w522] -> w505
          tunnel: w509 -> [w513 w521]
          tunnel: [w513 w521] -> w508
          frame True {
          }
          frame False {
            n243 = call "color-red-2.vi"("url"=w518, "error in (no error)"=w520, "client handle"=w519) -> ("error out"=w516:errorcluster, "client handle out"=w517:T9)  [unwired: 7 in]
            n244 = while {
              tunnel: w518 -> [w529]
              tunnel: w517 -> [w528]
              tunnel: w516 -> [w527]
              tunnel: [w525] -> w523
              tunnel: [w524] -> w522
              stop <- w526 continue-if-true
              n245 = call "is_moving.vi"("string"=w529, "error in (no error)"=w527, "client handle"=w528) -> ("error out"=w524:errorcluster, "moving"=w526:bool, "client handle out"=w525:T9)  [unwired: 6 in]
            }
          }
        }
      }
      frame True {
        n246 = call "color-green.vi"("url"=w537, "error in (no error)"=w533, "client handle"=w532) -> ("error out"=w539:errorcluster, "client handle out"=w538:T9)  [unwired: 7 in]
        n247 = call "is_paused.vi"("url"=w537, "error in (no error)"=w539, "client handle"=w538) -> ("error out"=w541:errorcluster, "paused"=w540:bool, "client handle out"=w542:T9)  [unwired: 6 in]
        n248 = case shown="False" w540 {
          tunnel: w534 -> [_ w550]
          tunnel: w536 -> [w543 w552]
          tunnel: w537 -> [_ w555]
          tunnel: w541 -> [w544 w557]
          tunnel: w542 -> [w545 w556]
          tunnel: [w543 w548] -> w535
          tunnel: [w545 w547] -> w531
          tunnel: [w544 w546] -> w530
          frame True {
          }
          frame False {
            n249 = Array Size(array=w550) -> (size(s)=w549:i32)
            n250 = Index Array(array=w550, index=w552) -> (element=w558:T10)
            n251 = Increment(x=w552) -> (x+1=w551:i32)
            n252 = Quotient & Remainder(x=w551, y=w549) -> (x-y*floor(x/y)=w548:i32)  [unwired: 1 out]
            n253 = call "send_angles.vi"("url"=w555, "error in (no error)"=w557, "angles and speed"=w558, "client handle"=w556) -> ("error out"=w553:errorcluster, "client handle out"=w554:T9)  [unwired: 6 in]
            n254 = while {
              tunnel: w555 -> [w564]
              tunnel: w554 -> [w563]
              tunnel: w553 -> [w562]
              tunnel: [w560] -> w547
              tunnel: [w559] -> w546
              stop <- w561 continue-if-true
              n255 = call "is_moving.vi"("string"=w564, "error in (no error)"=w562, "client handle"=w563) -> ("error out"=w559:errorcluster, "moving"=w561:bool, "client handle out"=w560:T9)  [unwired: 6 in]
            }
          }
        }
      }
    }
  }
  n256 = while {
    tunnel: w9 -> [w580]
    tunnel: w8 -> [w579]
    tunnel: w7 -> [w578]
    tunnel: [w577] -> w12
    tunnel: [w576] -> w5
    shift-right: [w574] -> _
    shift-left: 0 -> [w575]
    tunnel: "Threshold" -> [w569]
    stop <- FALSE stop-if-true
    n257 = local read "Channel"() -> (w566:bool)
    n258 = Not(x=w566) -> (.not. x?=w565:bool)
    n259 = local read "Switch mode"() -> (w567:bool)
    n260 = case shown="True" w565 {
      tunnel: [w581 w583] -> w568
      tunnel: w567 -> [_ w582]
      frame False {
        n261 = local read "BER HP3"() -> (w581:dbl)
      }
      frame True {
        n262 = case shown="True" w582 {
          tunnel: [w584 w585] -> w583
          frame False {
            n263 = local read "HP - CH0"() -> (w584:dbl)
          }
          frame True {
            n264 = local read "HP - CH0"() -> (w585:dbl)
          }
        }
      }
    }
    n265 = Wait (ms)(milliseconds to wait=u32 300) -> ()  [unwired: 1 out]
    n266 = Less?(x=w568, y=w569) -> (x < y?=w572:bool)
    n267 = case shown="False" w572 {
      tunnel: w580 -> [_ w623]
      tunnel: w575 -> [w590 w614]
      tunnel: w579 -> [w591 w615]
      tunnel: w578 -> [w592 w616]
      tunnel: [w588 w622] -> w577
      tunnel: [w587 w621] -> w576
      tunnel: [w589 w619] -> w574
      tunnel: "url" -> [w586 w613]
      frame False {
        n268 = call "is_paused.vi"("url"=w586, "error in (no error)"=w591, "client handle"=w592) -> ("error out"=w594:errorcluster, "paused"=w593:bool, "client handle out"=w595:T9)  [unwired: 6 in]
        n269 = case shown="False" w593 {
          tunnel: w586 -> [_ w599]
          tunnel: w594 -> [w597 w601]
          tunnel: w595 -> [w598 w600]
          tunnel: [w598 w606] -> w588
          tunnel: [w597 w605] -> w587
          tunnel: w590 -> [w596 w604]
          tunnel: [w596 w604] -> w589
          frame True {
          }
          frame False {
            n270 = call "color-red.vi"("url"=w599, "error in (no error)"=w601, "client handle"=w600) -> ("error out"=w602:errorcluster, "client handle out"=w603:T9)  [unwired: 7 in]
            n271 = while {
              tunnel: w599 -> [w612]
              tunnel: w603 -> [w611]
              tunnel: w602 -> [w610]
              tunnel: [w608] -> w606
              tunnel: [w607] -> w605
              stop <- w609 continue-if-true
              n272 = call "is_moving.vi"("string"=w612, "error in (no error)"=w610, "client handle"=w611) -> ("error out"=w607:errorcluster, "moving"=w609:bool, "client handle out"=w608:T9)  [unwired: 6 in]
            }
          }
        }
      }
      frame True {
        n273 = call "color-green.vi"("url"=w613, "error in (no error)"=w615, "client handle"=w616) -> ("error out"=w618:errorcluster, "client handle out"=w617:T9)  [unwired: 7 in]
        n274 = call "is_paused.vi"("url"=w613, "error in (no error)"=w618, "client handle"=w617) -> ("error out"=w624:errorcluster, "paused"=w620:bool, "client handle out"=w625:T9)  [unwired: 6 in]
        n275 = case shown="False" w620 {
          tunnel: w623 -> [_ w633]
          tunnel: w614 -> [w626 w635]
          tunnel: w613 -> [_ w638]
          tunnel: w624 -> [w627 w640]
          tunnel: w625 -> [w628 w639]
          tunnel: [w626 w631] -> w619
          tunnel: [w628 w630] -> w622
          tunnel: [w627 w629] -> w621
          frame True {
          }
          frame False {
            n276 = Array Size(array=w633) -> (size(s)=w632:i32)
            n277 = Index Array(array=w633, index=w635) -> (element=w641:T10)
            n278 = Increment(x=w635) -> (x+1=w634:i32)
            n279 = Quotient & Remainder(x=w634, y=w632) -> (x-y*floor(x/y)=w631:i32)  [unwired: 1 out]
            n280 = call "send_angles.vi"("url"=w638, "error in (no error)"=w640, "angles and speed"=w641, "client handle"=w639) -> ("error out"=w636:errorcluster, "client handle out"=w637:T9)  [unwired: 6 in]
            n281 = while {
              tunnel: w638 -> [w647]
              tunnel: w637 -> [w646]
              tunnel: w636 -> [w645]
              tunnel: [w643] -> w630
              tunnel: [w642] -> w629
              stop <- w644 continue-if-true
              n282 = call "is_moving.vi"("string"=w647, "error in (no error)"=w645, "client handle"=w646) -> ("error out"=w642:errorcluster, "moving"=w644:bool, "client handle out"=w643:T9)  [unwired: 6 in]
            }
          }
        }
      }
    }
  }
  n283 = call <vilib>:"CloseHandle.vi"("client handle"=w6, "error in (no error)"=w4) -> ()  [unwired: 13 in, 1 out]
  n284 = call <vilib>:"CloseHandle.vi"("client handle"=w12, "error in (no error)"=w5) -> ()  [unwired: 13 in, 1 out]
  n285 = Close File(refnum=w34, error in=w35) -> (error out=w38:errorcluster)  [unwired: 1 out]
  n286 = Close File(refnum=w16, error in=w15) -> (error out=w22:errorcluster)  [unwired: 1 out]
  n287 = Close File(refnum=w14, error in=w13) -> (error out=w21:errorcluster)  [unwired: 1 out]
  n288 = local read "iterationsIM"() -> (→"iterationsIM":dbl)
  n289 = call <vilib>:"Simple Error Handler.vi"("error in (no error)"=w38) -> ()  [unwired: 1 in, 8 out]
  n290 = call <vilib>:"Simple Error Handler.vi"("error in (no error)"=w22) -> ()  [unwired: 1 in, 8 out]
  n291 = call <vilib>:"Simple Error Handler.vi"("error in (no error)"=w21) -> ()  [unwired: 1 in, 8 out]
  n292 = call <instrlib>:"niUSRP Close Session.vi"("session handle"=w48, "error in (no error)"=w49) -> ()  [unwired: 13 in, 1 out]
  "No. Bits LP - CH0" <- w45
  "No. Bits - CH1" <- w45
  "No. Bits HP - CH0" <- w45
